vi "Initialize SysCfg Device.vi"(8 "error in":errorcluster, 9 "NI Auth":cluster{"User Name":string, "Password":string}[](array[cluster]), 10 "Target Address":string, 11 "Controller in":refnum<class "Controller.lvclass">) -> (0 "error out":errorcluster, 3 "Controller out":refnum<class "Controller.lvclass">)   [LabVIEW 2015, in "SMI.lvlib" / "SysCfg Device.lvclass"]
uses:
  SysCfg Device.lvclass
  Controller/Controller.lvclass
  SysCfg Device.lvclass/SysCfg Device.ctl
  Accessor Methods/Write User Name.vi
  Accessor Methods/Write Password.vi
  Write SysCfg Session.vi
  <vilib>/nisyscfg/Close (System).vi
  <vilib>/nisyscfg/nisyscfg.lvlib
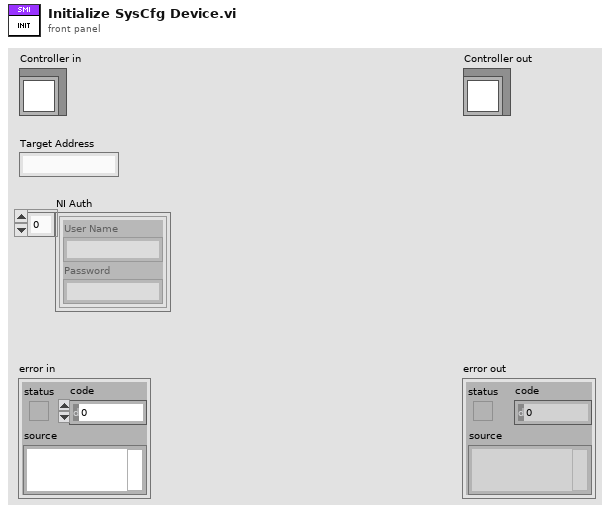
[diagram p1: front panel]
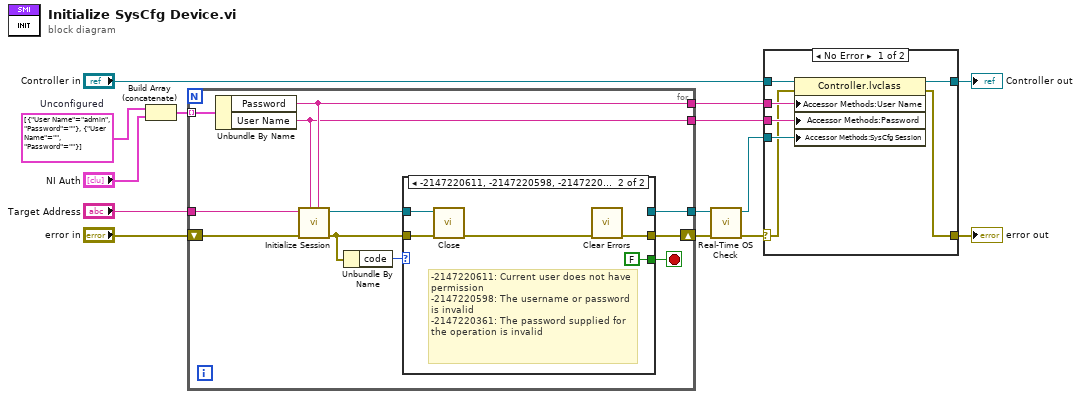
[diagram p0: block diagram]
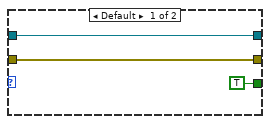
[diagram p3: hidden frame]
diagram:
  w8 = cluster{"User Name":string, "Password":string}[] [{"User Name"="admin", "Password"=""}, {"User Name"="", "Password"=""}]  # Unconfigured
  n1 = Build Array (concatenate)(w8, "NI Auth") -> (w9:cluster{"User Name":string, "Password":string}[])
  n2 = for {
    tunnel: "Target Address" -> [w25]
    shift-right: [w17] -> w5
    shift-left: "error in" -> [w24]
    tunnel: w9 -> [w23] mode=indexing
    tunnel: [w18] -> w3
    tunnel: [w16] -> w7
    tunnel: [w15] -> w6
    stop <- w19 stop-if-true
    n3 = Unbundle By Name(w23) -> ("Password"=w16:string, "User Name"=w15:string)
    n4 = call <vilib>:"Initialize Session.vi"("Password"=w16, "User Name"=w15, "error in (no error)"=w24, "Target (localhost)"=w25) -> ("error out"=w21:errorcluster, "Session out"=w20:refnum<k21>)  [unwired: 6 in]
    n5 = Unbundle By Name(w21) -> ("code"=w22:i32)
    n6 = case shown="-2147220611, -2147220598, -2147220361" w22 {
      tunnel: w20 -> [w28 w29]
      tunnel: w21 -> [w27 w33]
      tunnel: [w27 w30] -> w17
      tunnel: [w28 _] -> w18
      tunnel: [TRUE FALSE] -> w19
      frame Default {
      }
      frame -2147220611, -2147220598, -2147220361 {
        # "-2147220611: Current user does not have permission\n-2147220598: The username or password is invalid \n-2147220361: The password supplied for the operation is invalid"
        n7 = call-poly <vilib>:"Close.vi"("error in (no error)"=w33, "Session in"=w29) -> ("error out"=w31:errorcluster)  [unwired: 9 in]
        n8 = call <vilib>:"Clear Errors.vi"("error in (no error)"=w31) -> ("error out"=w30:errorcluster)  [unwired: 5 in, 1 out]
      }
    }
  }
  n9 = call "Real-Time OS Check.vi"("error in"=w5, "System Session in"=w3) -> ("error out"=w2:errorcluster, "System Session out"=w4:refnum<k21>)  [unwired: 8 in]
  n10 = case shown="No Error" w2 {
    selector: w2 -> [w35 w42]
    tunnel: "Controller in" -> [w40 w41]
    tunnel: [w39 w41] -> w12
    tunnel: w7 -> [w38 _]
    tunnel: w6 -> [w37 _]
    tunnel: w4 -> [w36 _]
    tunnel: [w34 w42] -> w1
    frame No Error {
      n11 = property class="Controller.lvclass"(reference=w40, error in=w35, "Accessor Methods:User Name"=w38, "Accessor Methods:Password"=w37, "Accessor Methods:SysCfg Session"=w36) -> (reference out=w39:refnum<class "Controller.lvclass">, error out=w34:errorcluster)
    }
    frame Error {
    }
  }
  "error out" <- w1
  "Controller out" <- w12
